vi "niSwitch Detach gRPC Session.vi"(8 "error in":errorcluster, 11 "session factory in":refnum<class "Session Factory.lvclass">) -> (0 "error out":errorcluster)   [LabVIEW 2021, in "Session Management niSwitch.lvlib" / "Session Factory.lvclass"]
doc: "Detaches from the gRPC session specified in <b>session factory in</b>."
uses:
  Session Factory.lvclass
  Session Factory.lvclass/Session Factory.ctl
  NI Switch Client/NI Switch Client.lvlib
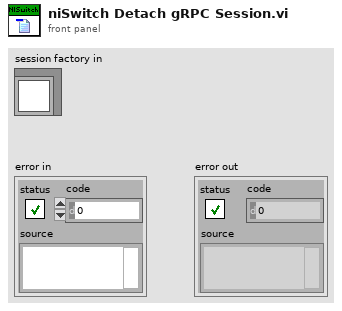
[diagram p1: front panel]
types:
  T1 = typedef "grpc-lvsupport-release.lvlib/grpcId.ctl" = u64
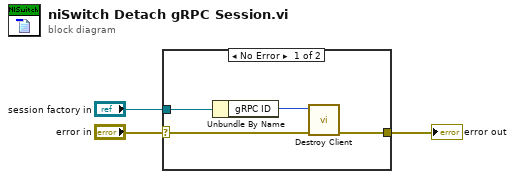
[diagram p0: block diagram]
diagram:
  n1 = case shown="No Error" "error in" {
    selector: "error in" -> [w7 w8]
    tunnel: [w6 w8] -> w1
    tunnel: "session factory in" -> [w4 _]
    frame No Error {
      n2 = Unbundle By Name(w4) -> ("gRPC ID"=w5:T1)
      n3 = call "Destroy Client.vi"("error in"=w7, "gRPC ID"=w5) -> ("error out"=w6:errorcluster)  [unwired: 9 in]
    }
    frame Error {
    }
  }
  "error out" <- w1
